vi "ToRepo.vi"(8 "error in":errorcluster, 9 "to repo cluster":T1, 10 "repository in":refnum<class "NISE_CEF_Repository.lvclass">, 11 "SequenceNode in":refnum<class "SequenceNode.lvclass">) -> (0 "error out":errorcluster, 2 "repository out":refnum<class "NISE_CEF_Repository.lvclass">, 3 "SequenceNode out":refnum<class "SequenceNode.lvclass">)   [LabVIEW 2015, in "SequenceNode.lvclass"]
doc: "Copyright 2017 National Instruments Corporation\n\nLicensed under the Apache License, Version 2.0 (the \"License\"); you may not use this file except in compliance with the License. You may obtain a copy of the License at http://www.apache.org/licenses/LICENSE-2.0\nUnless required by applicable law or agreed to in writing, software distributed under the License is distributed on an \"AS IS\" BASIS, WITHOUT WARRANTIES OR CONDITIONS OF ANY KIND, either express or implied. See the License for the specific language governing permissions and limitations under the License."
uses:
  SequenceNode.lvclass
  <vilib>/NI/Configuration Framework/Repository/NISE_CEF_Repository.lvclass
  <vilib>/NI/Configuration Framework/Node/ToRepoCluster.ctl
  SequenceRepo/SequenceRepo.lvclass
  Prototype/classes/Sequence/Config/Sequence Config.lvclass
  <vilib>/NI/Configuration Framework/Node/NISE_CEF_Node.lvclass
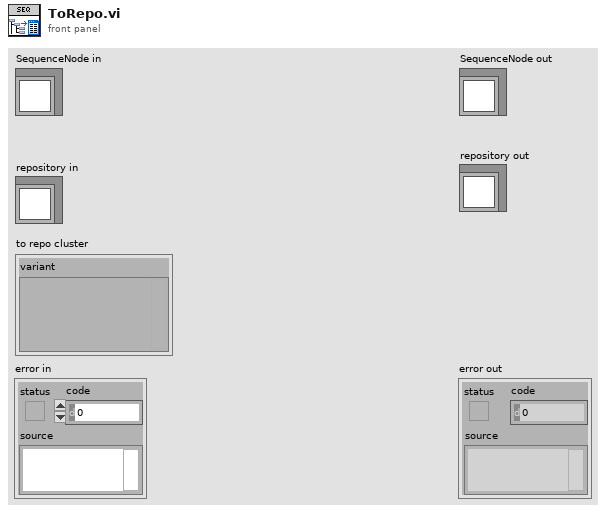
[diagram p1: front panel]
types:
  T1 = typedef "NISE_CEF_Node.lvclass/ToRepoCluster.ctl" = cluster{"variant":variant}
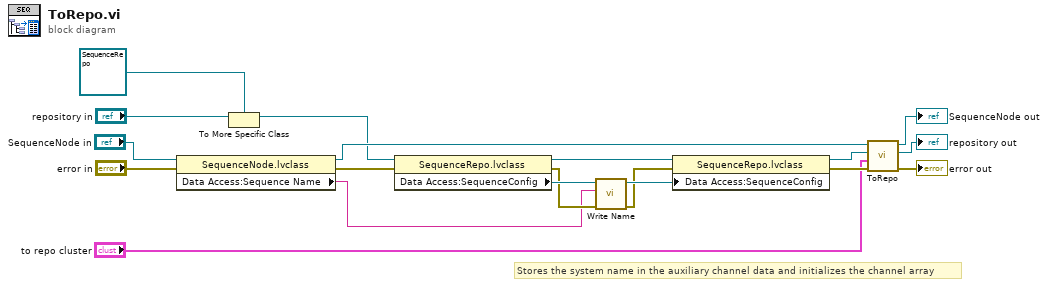
[diagram p0: block diagram]
diagram:
  # "Stores the system name in the auxiliary channel data and initializes the channel array"
  n1 = property class="SequenceNode.lvclass"(reference="SequenceNode in", error in="error in") -> (reference out=w12:refnum<class "SequenceNode.lvclass">, error out=w10:errorcluster, "Data Access:Sequence Name"=w1:string)
  n2 = To More Specific Class(target class=refnum<class "SequenceRepo.lvclass"> refnum ("cRIO repo.lvclass"), reference="repository in") -> (specific class reference=w7:refnum<class "SequenceRepo.lvclass">)  [unwired: 1 in, 1 out]
  n3 = property class="SequenceRepo.lvclass"(reference=w7, error in=w10) -> (reference out=w6:refnum<class "SequenceRepo.lvclass">, error out=w3:errorcluster, "Data Access:SequenceConfig"=w5:refnum<class "Sequence Config.lvclass">)
  n4 = call-dynamic "Write Name.vi"("error in (no error)"=w3, "Name"=w1, "Sequence in"=w5) -> ("error out"=w2:errorcluster, "Sequence out"=w4:refnum<class "Sequence Config.lvclass">)  [unwired: 7 in]
  n5 = property class="SequenceRepo.lvclass"(reference=w6, error in=w2, "Data Access:SequenceConfig"=w4) -> (reference out=w16:refnum<class "SequenceRepo.lvclass">, error out=w9:errorcluster)
  n6 = call-parent "ToRepo.vi"("error in"=w9, "to repo cluster"="to repo cluster", "repository in"=w16, "node in"=w12) -> ("error out"=→"error out":errorcluster, "repository out"=→"repository out":refnum<class "NISE_CEF_Repository.lvclass">, "node out"=→"SequenceNode out":refnum<class "SequenceNode.lvclass">)  [unwired: 5 in]
